vi "MathCad_Matrix_Set_Elmnt.vi"(0 "Worksheet Reference In":refnum<k7>, 2 "value":dbl format="%.2f", 5 "Mathcad.IMatrixValue":refnum<k7>, 7 "row":i32, 9 "col":i32, 11 "error in":errorcluster) -> (4 "Worksheet Reference Out":refnum<k7>, 6 "Mathcad.IMatrixValue Refnum out":refnum<k7>, 15 "error out":errorcluster)   [LabVIEW 2015]
doc: "Sets the value of the reference. This must be done before inserting into a worksheet."
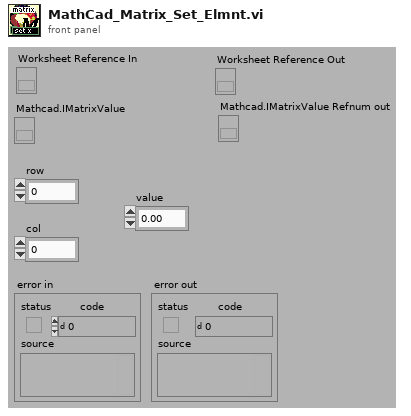
[diagram p1: front panel]
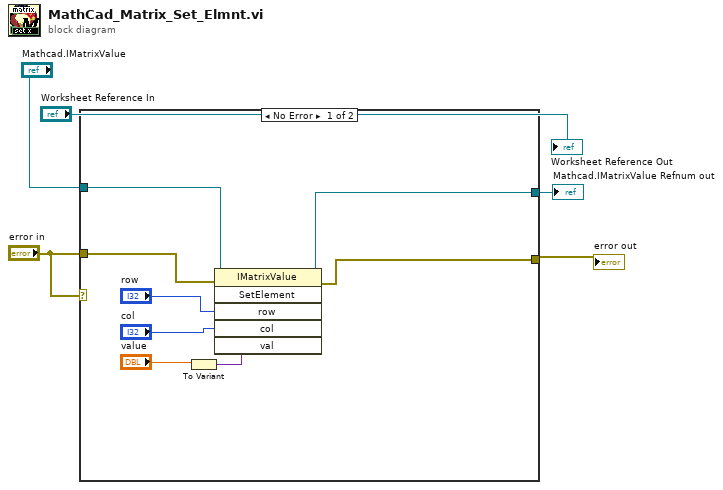
[diagram p0: block diagram]
diagram:
  n1 = case shown="No Error" "error in" {
    tunnel: "error in" -> [w10 w15]
    tunnel: [w7 w15] -> w5
    tunnel: "Mathcad.IMatrixValue" -> [w6 w14]
    tunnel: [w13 w14] -> w1
    frame No Error {
      n2 = To Variant(anything="value") -> (Variant=w9:variant)
      n3 = invoke class="IMatrixValue" method="SetElement"(reference=w6, error in=w10, "row"="row", "col"="col", "val"=w9) -> (reference out=w13:refnum<k7>, error out=w7:errorcluster)  [unwired: 1 in, 4 out]
    }
    frame Error {
    }
  }
  "error out" <- w5
  "Mathcad.IMatrixValue Refnum out" <- w1
  "Worksheet Reference Out" <- "Worksheet Reference In"
